vi "RetrieveDefaultDotData.vi"(8 "error in (no error)":errorcluster, 10 "Path":path, 11 "Setting Database In":refnum<class "Setting Database.lvclass">) -> (0 "error out":errorcluster, 2 "Dot Settings out":refnum<class "Dot Settings.lvclass">, 3 "Setting Database Out":refnum<class "Setting Database.lvclass">)   [LabVIEW 2019, in "Setting Database.lvclass"]
uses:
  Setting Database.lvclass
  Dot Settings/Dot Settings.lvclass
  Setting Database.lvclass/Setting Database.ctl
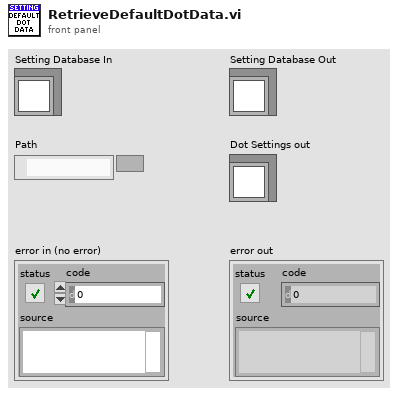
[diagram p1: front panel]
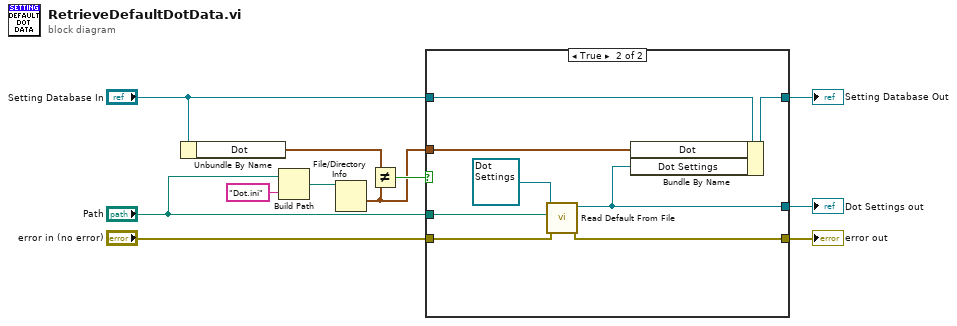
[diagram p0: block diagram]
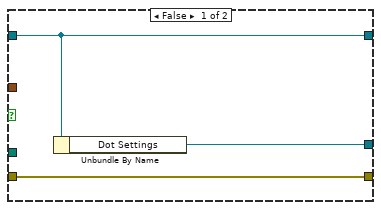
[diagram p2: hidden frame]
diagram:
  n1 = Unbundle By Name("Setting Database In") -> ("Dot"=w2:timestamp)
  n2 = Build Path(base path="Path", name or relative path="Dot.ini") -> (appended path=w7:path)
  n3 = File/Directory Info(path=w7) -> (last mod=w1:timestamp)  [unwired: 1 in, 6 out]
  n4 = Not Equal?(x=w2, y=w1) -> (x != y?=w5:bool)
  n5 = case shown="True" w5 {
    tunnel: [w14 w17] -> w10
    tunnel: "Path" -> [_ w22]
    tunnel: "Setting Database In" -> [w13 w20]
    tunnel: [w13 w21] -> w11
    tunnel: "error in (no error)" -> [w12 w18]
    tunnel: [w12 w19] -> w9
    tunnel: w1 -> [_ w15]
    frame False {
      n6 = Unbundle By Name(w13) -> ("Dot Settings"=w14:refnum<class "Dot Settings.lvclass">)
    }
    frame True {
      n7 = call-dynamic "Read Default From File.vi"("error in (no error)"=w18, "Path"=w22, "Dot Settings in"=refnum<class "Dot Settings.lvclass"> refnum ("Dot Settings.lvclass")) -> ("error out"=w19:errorcluster, "Dot Settings out"=w17:refnum<class "Dot Settings.lvclass">)  [unwired: 7 in]
      n8 = Bundle By Name(cluster=w20, "Dot"=w15, "Dot Settings"=w17) -> (w21:refnum<class "Setting Database.lvclass">)
    }
  }
  "error out" <- w9
  "Dot Settings out" <- w10
  "Setting Database Out" <- w11
